vi "Waveform.Selection.vi"(8 "error in (no error)":errorcluster, 11 "NewVal":path) -> (0 "error out":errorcluster, 2 "Apply?":bool, 3 "Data":waveform(dbl)[](array[waveform]))   [LabVIEW 2019, in "Fuel Injector Analysis Addon System Explorer.lvlib"]
uses:
  Fuel Injector Analysis Addon System Explorer.lvlib
panel:
  in  "Cancel":bool
  in  "Apply":bool
  in  "Current Channel":string(combo)
  in  "Voltage Channel":string(combo)
  out "Injection":waveform(dbl)[](graph)
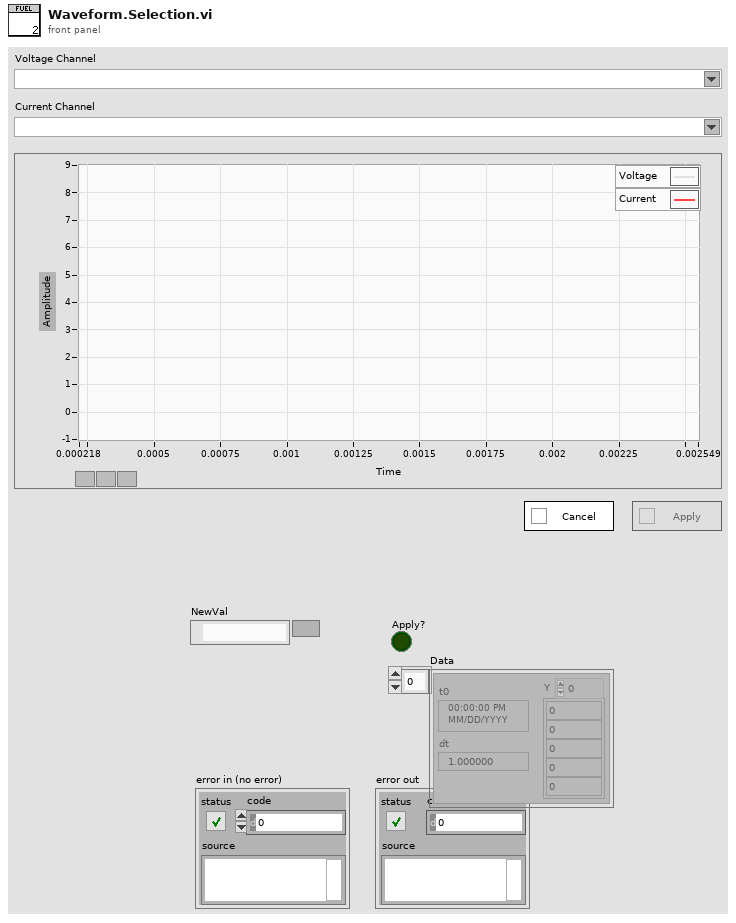
[diagram p1: front panel]
types:
  T1 = enum8{"Enabled", "Disabled", "Disabled and Grayed Out"}
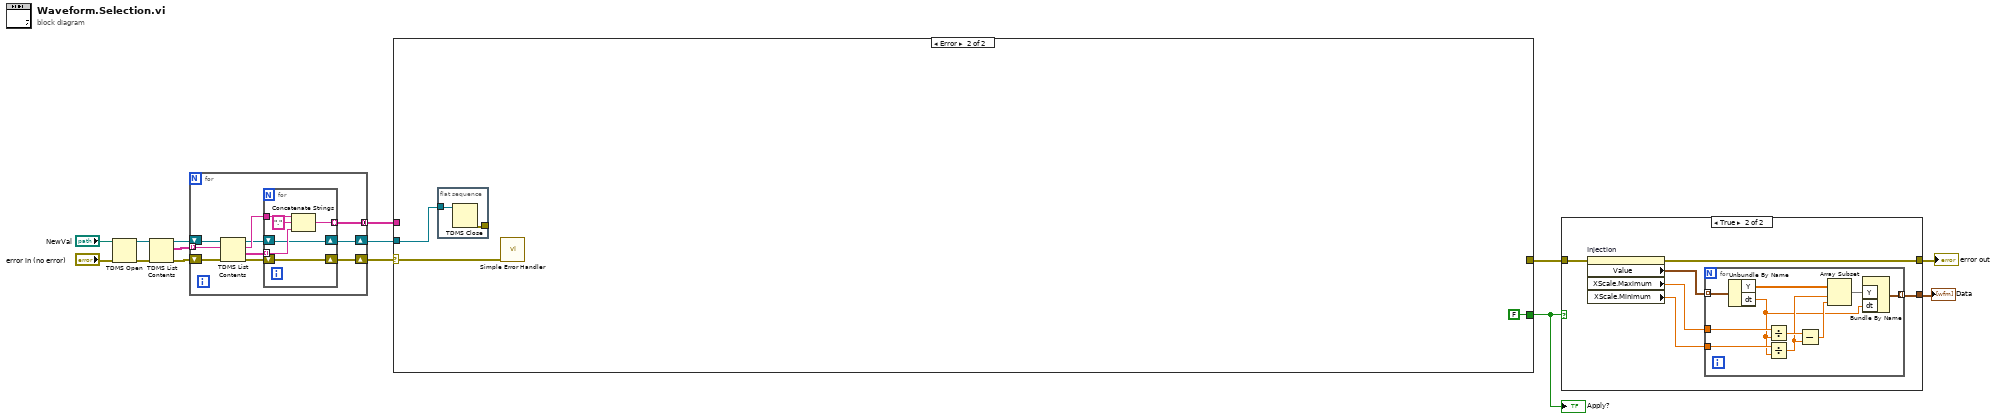
[diagram p0: block diagram]
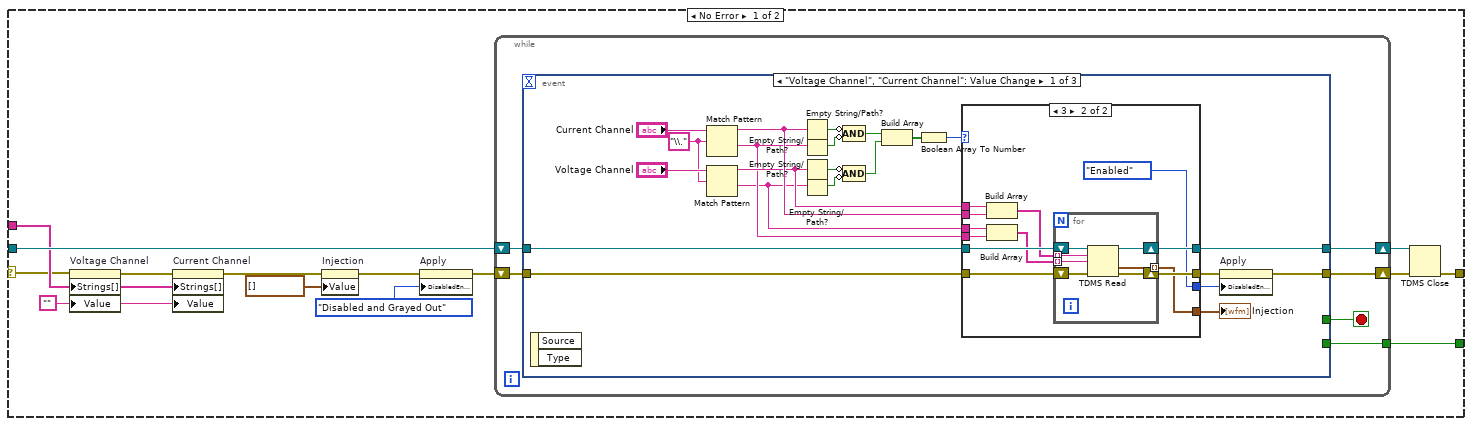
[diagram p2: hidden frame]
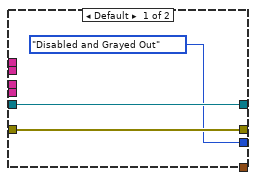
[diagram p3: hidden frame]
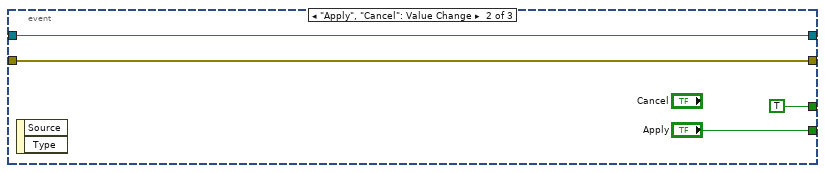
[diagram p4: hidden frame]
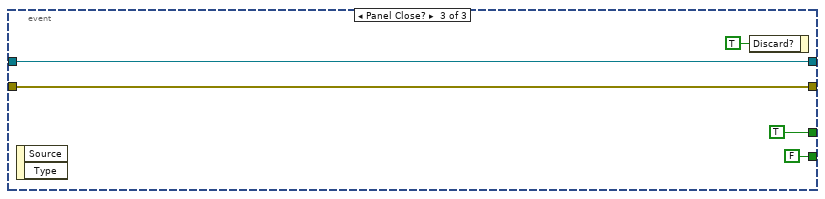
[diagram p5: hidden frame]
diagram:
  n1 = TDMS Open(8:"error in (no error)", 11:"NewVal") -> (0:w10:errorcluster, 3:w11:refnum<k34>)  [unwired: 5 in]
  n2 = TDMS List Contents(4:w10, 7:w11) -> (0:w12:errorcluster, 2:w7:string[], 3:w13:refnum<k34>)  [unwired: 1 in, 1 out]
  n3 = for {
    tunnel: w7 -> [w22] mode=indexing
    shift-right: [w16] -> w14
    shift-left: w13 -> [w24]
    shift-right: [w15] -> w1
    shift-left: w12 -> [w23]
    tunnel: [w17] -> w6 mode=concatenating
    n4 = TDMS List Contents(4:w23, 6:w22, 7:w24) -> (0:w20:errorcluster, 1:w18:string[], 2:w21:string, 3:w19:refnum<k34>)
    n5 = for {
      tunnel: w21 -> [w30]
      shift-right: [w26] -> w16
      shift-left: w19 -> [w26]
      shift-right: [w27] -> w15
      shift-left: w20 -> [w27]
      tunnel: w18 -> [w28] mode=indexing
      tunnel: [w25] -> w17 mode=indexing
      n6 = Concatenate Strings(w30, "." ("string"), w28) -> (w25:string)
    }
  }
  n7 = case shown="Error" w1 {
    selector: w1 -> [w31 w105]
    tunnel: w14 -> [w42 w104]
    tunnel: w6 -> [w40 _]
    tunnel: [w33 _] -> w5
    tunnel: [w32 FALSE ("Apply")] -> w2
    frame No Error {
      w37 = ""
      n8 = property on="Voltage Channel" class="CmbBox"(error in=w31, "Strings[]"=w40, "Value"=w37) -> (error out=w41:errorcluster)  [unwired: 1 in, 1 out]
      n9 = property on="Current Channel" class="CmbBox"(error in=w41, "Strings[]"=w40, "Value"=w37) -> (error out=w39:errorcluster)  [unwired: 1 in, 1 out]
      n10 = property on="Injection" class="WFGraph (strict)"(error in=w39, "Value"=waveform(dbl)[] [] ("Injection")) -> (error out=w36:errorcluster)  [unwired: 1 in, 1 out]
      n11 = property on="Apply" class="Bool"(error in=w36, "DisabledEnum"=T1."Disabled and Grayed Out" ("Disabled")) -> (error out=w35:errorcluster)  [unwired: 1 in, 1 out]
      n12 = while {
        shift-right: [w50] -> w44
        shift-left: w42 -> [w48]
        shift-right: [w49] -> w43
        shift-left: w35 -> [w47]
        tunnel: [w45] -> w32
        stop <- w46 stop-if-true
        n13 = event shown="[0] \"Voltage Channel\", \"Current Channel\": Value Change" {
          selector: _ -> [_ _ _]
          dyn-events: _ -> [_ _ _]
          timeout: _ -> [_ _ _]
          tunnel: [w72 w97 w102] -> w50
          tunnel: [w52 w98 w103] -> w49
          tunnel: w48 -> [w71 w97 w102]
          tunnel: w47 -> [w70 w98 w103]
          tunnel: [_ TRUE TRUE] -> w46
          tunnel: [_ "Apply" FALSE ("Apply")] -> w45
          event "Voltage Channel", "Current Channel": Value Change {
            w67 = "\\." ("regular expression")
            n14 = event-data() -> ()  [unwired: 1 in, 2 out]
            n15 = Match Pattern(string="Current Channel", regular expression=w67) -> (before substring=w58:string, after substring=w56:string)  [unwired: 1 in, 2 out]
            n16 = Match Pattern(string="Voltage Channel", regular expression=w67) -> (before substring=w57:string, after substring=w55:string)  [unwired: 1 in, 2 out]
            n17 = Empty String/Path?(string/path=w58) -> (empty?=w66:bool)
            n18 = Empty String/Path?(string/path=w56) -> (empty?=w65:bool)
            n19 = Empty String/Path?(string/path=w57) -> (empty?=w63:bool)
            n20 = Empty String/Path?(string/path=w55) -> (empty?=w64:bool)
            n21 = Compound Arithmetic op=AND(invert w66, invert w65) -> (w62:bool)
            n22 = Compound Arithmetic op=AND(invert w63, invert w64) -> (w61:bool)
            n23 = Build Array(w62, w61) -> (w60:bool[])
            n24 = Boolean Array To Number(Boolean array=w60) -> (number=w59:u32)
            n25 = case shown="3" w59 {
              tunnel: [w74 w87] -> w72
              tunnel: [w75 w86] -> w53
              tunnel: w71 -> [w74 w85]
              tunnel: w70 -> [w75 w84]
              tunnel: w58 -> [_ w76]
              tunnel: w57 -> [_ w77]
              tunnel: w56 -> [_ w78]
              tunnel: w55 -> [_ w79]
              tunnel: [_ w83] -> w54
              tunnel: [T1."Disabled and Grayed Out" ("Disabled") T1."Enabled" ("Disabled")] -> w51
              frame Default {
              }
              frame 3 {
                n26 = Build Array(w77, w76) -> (w82:string[])
                n27 = Build Array(w79, w78) -> (w81:string[])
                n28 = for {
                  tunnel: [w90] -> w83 mode=indexing
                  tunnel: w82 -> [w89] mode=indexing
                  shift-right: [w94] -> w87
                  shift-left: w85 -> [w92]
                  shift-right: [w93] -> w86
                  shift-left: w84 -> [w91]
                  tunnel: w81 -> [w88] mode=indexing
                  n29 = TDMS Read(0:w92, 5:w89, 7:w88, 11:w91) -> (4:w94:refnum<k34>, 10:w90:waveform(dbl), 15:w93:errorcluster)  [unwired: 4 in, 3 out]
                }
              }
            }
            "Injection" <- w54
            n30 = property on="Apply" class="Bool"(error in=w53, "DisabledEnum"=w51) -> (error out=w52:errorcluster)  [unwired: 1 in, 1 out]
          }
          event "Apply", "Cancel": Value Change {
            n31 = event-data() -> ()  [unwired: 1 in, 2 out]
          }
          event Panel Close? {
            n32 = event-data() -> ()  [unwired: 1 in, 2 out]
            n33 = event-data("Discard?"=TRUE) -> ()  [unwired: 1 in, 1 out]
          }
        }
      }
      n34 = TDMS Close(8:w43, 11:w44) -> (0:w33:errorcluster)  [unwired: 1 out]
    }
    frame Error {
      n35 = flat-sequence {
        tunnel: w104 -> [w108]
        tunnel: [w107] -> _
        frame #0 {
          n36 = TDMS Close(11:w108) -> (0:w107:errorcluster)  [unwired: 1 in, 1 out]
        }
      }
      n37 = call <vilib>:"Simple Error Handler.vi"("error in (no error)"=w105) -> ()  [unwired: 4 in, 5 out]
    }
  }
  "Apply?" <- w2
  n38 = case shown="True" w2 {
    tunnel: w5 -> [w109 w112]
    tunnel: [w109 w111] -> w4
    tunnel: [_ w110] -> w3
    frame False {
    }
    frame True {
      n39 = property on="Injection" class="WFGraph (strict)"(error in=w112) -> (error out=w111:errorcluster, "Value"=w115:waveform(dbl)[], "XScale.Maximum"=w114:dbl, "XScale.Minimum"=w113:dbl)  [unwired: 1 in, 1 out]
      n40 = for {
        tunnel: w115 -> [w125] mode=indexing
        tunnel: w114 -> [w124]
        tunnel: w113 -> [w123]
        tunnel: [w116] -> w110 mode=indexing
        n41 = Unbundle By Name(w125) -> ("Y"=w121:dbl[], "dt"=w117:dbl)
        n42 = Divide(x=w124, y=w117) -> (x/y=w122:dbl)
        n43 = Divide(x=w123, y=w117) -> (x/y=w120:dbl)
        n44 = Subtract(x=w122, y=w120) -> (x-y=w119:dbl)
        n45 = Array Subset(array=w121, index=w120, length=w119) -> (w118:dbl[])
        n46 = Bundle By Name("Y"=w118, "dt"=w117) -> (w116:waveform(dbl))  [unwired: 1 in]
      }
    }
  }
  "error out" <- w4
  "Data" <- w3
